vi "Add Library To Project.vi"(8 "error in":errorcluster, 10 "library path":path, 11 "configuration":T1) -> (0 "error out":errorcluster, 3 "project ref out":refnum<vi>)   [LabVIEW 2021, in "InstrumentStudio Plug-In Editor.lvlib"]
uses:
  InstrumentStudio Plug-In Editor.lvlib
  controls/Data Holder.ctl
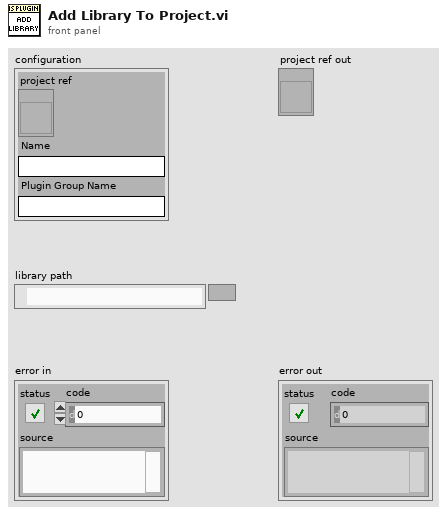
[diagram p1: front panel]
types:
  T1 = typedef "InstrumentStudio Plug-In Editor.lvlib/Data Holder.ctl" = cluster{"project ref":refnum<vi>, "Name":string, "Plugin Group Name":string}
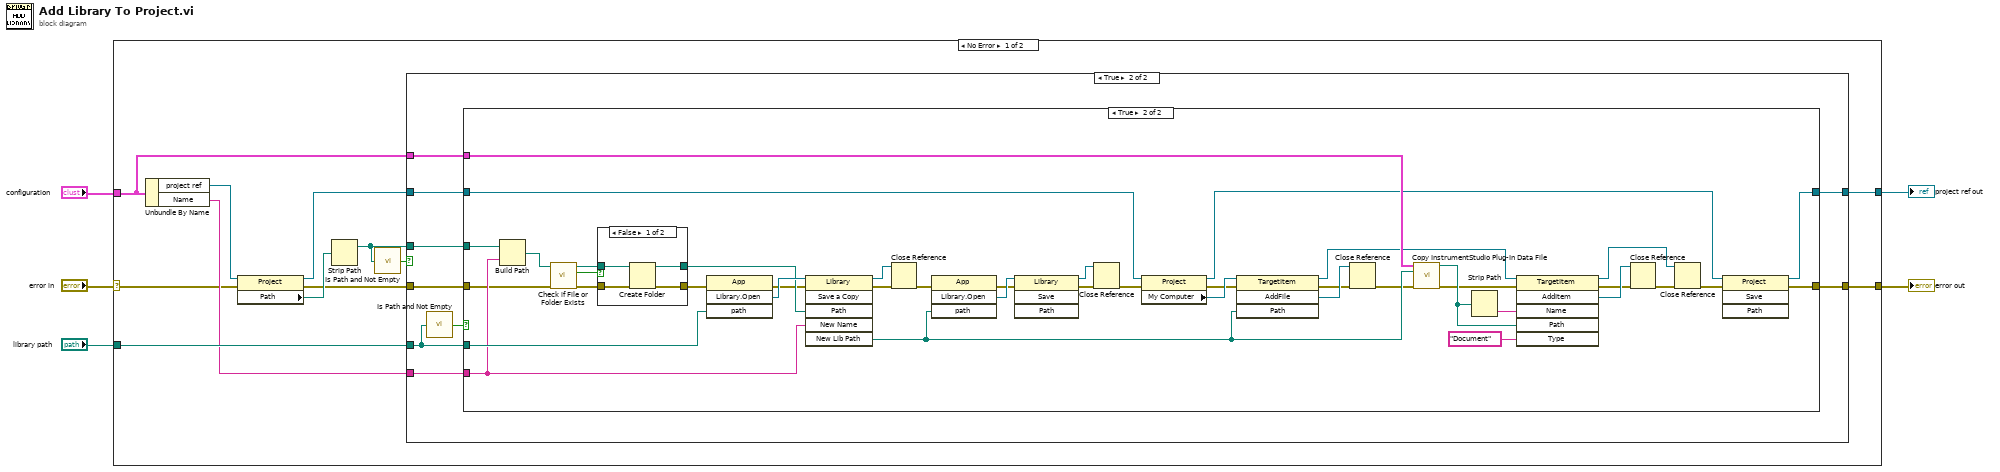
[diagram p0: block diagram]
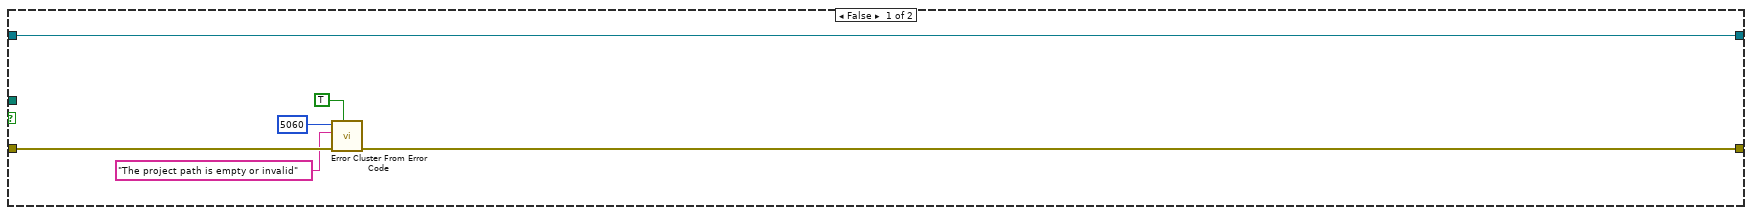
[diagram p2: hidden frame]
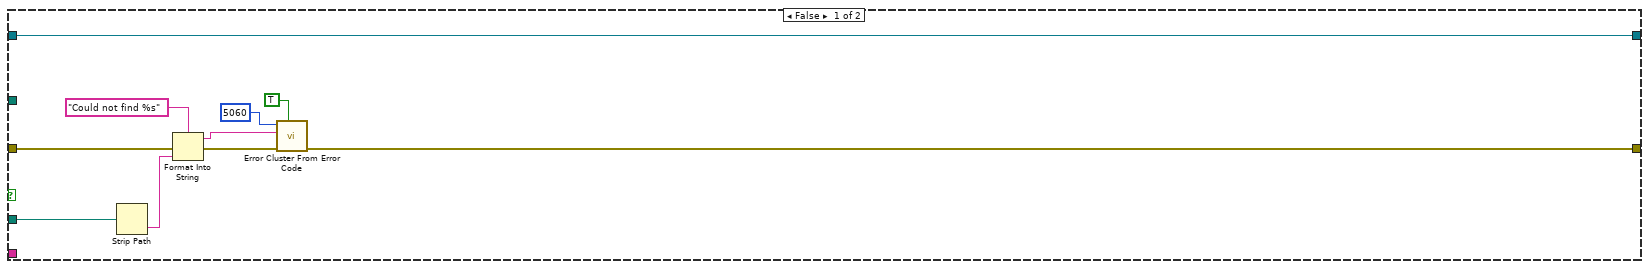
[diagram p3: hidden frame]
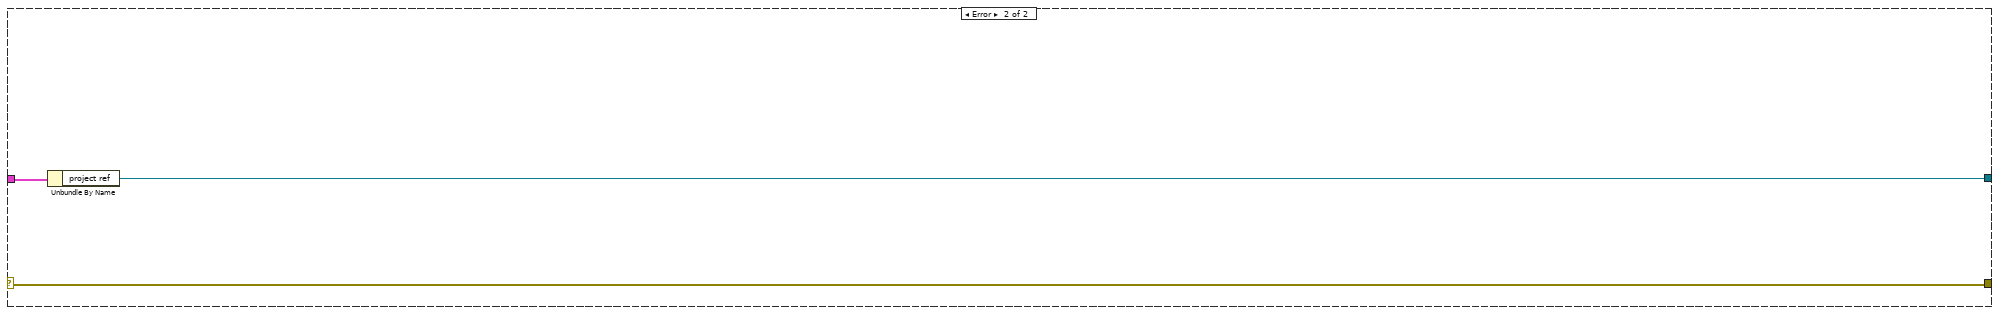
[diagram p5: hidden frame]
diagram:
  n1 = case shown="No Error" "error in" {
    selector: "error in" -> [w8 w91]
    tunnel: "library path" -> [w15 _]
    tunnel: [w14 w92] -> w3
    tunnel: "configuration" -> [w11 w90]
    tunnel: [w6 w91] -> w1
    frame No Error {
      n2 = Unbundle By Name(w11) -> ("project ref"=w13:refnum<vi>, "Name"=w12:string)
      n3 = property class="Project"(reference=w13, error in=w8) -> (reference out=w10:refnum<vi>, error out=w7:errorcluster, "Path"=w16:path)
      n4 = Strip Path(path=w16) -> (stripped path=w9:path)  [unwired: 1 out]
      n5 = call <vilib>:"Is Path and Not Empty.vi"("path"=w9) -> ("Is Path and Not Empty?"=w17:bool)  [unwired: 4 in]
      n6 = case shown="True" w17 {
        tunnel: w15 -> [_ w24]
        tunnel: w12 -> [_ w32]
        tunnel: w9 -> [_ w31]
        tunnel: [w23 w30] -> w14
        tunnel: w11 -> [_ w29]
        tunnel: w10 -> [w23 w28]
        tunnel: w7 -> [w22 w26]
        tunnel: [w18 w25] -> w6
        frame False {
          n7 = call <vilib>:"Error Cluster From Error Code.vi"("show call chain? (False)"=TRUE, "error in (no error)"=w22, "error message (\"\")"="The project path is empty or invalid" ("error message (\"\")"), "error code (0)"=5060) -> ("error out"=w18:errorcluster)  [unwired: 5 in]
        }
        frame True {
          n8 = call <vilib>:"Is Path and Not Empty.vi"("path"=w24) -> ("Is Path and Not Empty?"=w27:bool)  [unwired: 4 in]
          n9 = case shown="True" w27 {
            tunnel: w24 -> [w38 w83]
            tunnel: w32 -> [_ w80]
            tunnel: w31 -> [_ w82]
            tunnel: [w40 w74] -> w30
            tunnel: w29 -> [_ w72]
            tunnel: w28 -> [w40 w67]
            tunnel: w26 -> [w36 w62]
            tunnel: [w33 w43] -> w25
            frame False {
              n10 = Strip Path(path=w38) -> (name=w37:string)  [unwired: 1 out]
              n11 = Format Into String(format string="Could not find %s", error in=w36, w37) -> (resulting string=w41:string, error out=w42:errorcluster)  [unwired: 1 in]
              n12 = call <vilib>:"Error Cluster From Error Code.vi"("show call chain? (False)"=TRUE, "error in (no error)"=w42, "error message (\"\")"=w41, "error code (0)"=5060) -> ("error out"=w33:errorcluster)  [unwired: 5 in]
            }
            frame True {
              n13 = Build Path(base path=w82, name or relative path=w80) -> (appended path=w81:path)
              n14 = call <vilib>:"Check if File or Folder Exists.vi"("error in (no error)"=w62, "path"=w81) -> ("error out"=w61:errorcluster, "file or folder exists?"=w59:bool, "dup path"=w60:path)  [unwired: 7 in]
              n15 = case shown="False" w59 {
                tunnel: w61 -> [w87 w88]
                tunnel: w60 -> [w86 w89]
                tunnel: [w85 w89] -> w58
                tunnel: [w84 w88] -> w57
                frame False {
                  n16 = Create Folder(path (use dialog)=w86, error in=w87) -> (created path=w85:path, error out=w84:errorcluster)  [unwired: 1 in, 1 out]
                }
                frame True {
                }
              }
              n17 = invoke class="App" method="Library.Open"(error in=w57, "path"=w83) -> (error out=w56:errorcluster, "Open Library"=w79:refnum<vi>)  [unwired: 2 in, 2 out]
              n18 = invoke class="Library" method="Save a Copy"(reference=w79, error in=w56, "Path"=w58, "New Name"=w80) -> (reference out=w77:refnum<vi>, error out=w55:errorcluster, "New Lib Path"=w73:path)  [unwired: 2 in, 3 out]
              n19 = Close Reference(reference=w77, error in (no error)=w55) -> (error out=w54:errorcluster)
              n20 = invoke class="App" method="Library.Open"(error in=w54, "path"=w73) -> (error out=w53:errorcluster, "Open Library"=w75:refnum<vi>)  [unwired: 2 in, 2 out]
              n21 = invoke class="Library" method="Save"(reference=w75, error in=w53) -> (reference out=w76:refnum<vi>, error out=w52:errorcluster)  [unwired: 2 in, 2 out]
              n22 = Close Reference(reference=w76, error in (no error)=w52) -> (error out=w51:errorcluster)
              n23 = property class="Project"(reference=w67, error in=w51) -> (reference out=w63:refnum<vi>, error out=w50:errorcluster, "My Computer"=w78:refnum<vi>)
              n24 = invoke class="TargetItem" method="AddFile"(reference=w78, error in=w50, "Path"=w73) -> (reference out=w69:refnum<vi>, error out=w49:errorcluster, "AddFile"=w70:refnum<vi>)  [unwired: 1 in, 1 out]
              n25 = Close Reference(reference=w70, error in (no error)=w49) -> (error out=w48:errorcluster)
              n26 = call "Copy InstrumentStudio Plug-In Data File.vi"("configuration"=w72, "Plugin Path"=w73, "error in"=w48) -> ("G Plugin Data File Path"=w71:path, "error out"=w47:errorcluster)  [unwired: 11 in]
              n27 = Strip Path(path=w71) -> (name=w66:string)  [unwired: 1 out]
              n28 = invoke class="TargetItem" method="AddItem"(reference=w69, error in=w47, "Name"=w66, "Path"=w71, "Type"="Document") -> (reference out=w64:refnum<vi>, error out=w44:errorcluster, "AddItem"=w68:refnum<vi>)  [unwired: 1 in, 3 out]
              n29 = Close Reference(reference=w68, error in (no error)=w44) -> (error out=w46:errorcluster)
              n30 = Close Reference(reference=w64, error in (no error)=w46) -> (error out=w45:errorcluster)
              n31 = invoke class="Project" method="Save"(reference=w63, error in=w45) -> (reference out=w74:refnum<vi>, error out=w43:errorcluster)  [unwired: 2 in, 2 out]
            }
          }
        }
      }
    }
    frame Error {
      n32 = Unbundle By Name(w90) -> ("project ref"=w92:refnum<vi>)
    }
  }
  "error out" <- w1
  "project ref out" <- w3
